vi "fgv_gloabal-config.vi"(7 "cmd":T4, 11 "config_aging":T1 {"Test Specs"."출력단 특성전류 Irms[mA]  Min" format="%#.2f"; "Test Specs"."출력단 특성 전류 Irms[mA]  Max" format="%#.2f"; "Test Specs"."출력단 단선 Irms[mA](이하)" format="%#.2f"; "Test Specs"."제어단 특성 전류 Irms[mA] Min" format="%#.2f"; "Test Specs"."제어단 특성 전류 Irms[mA] Max" format="%#.2f"; "Test Specs"."제어단 단선 Irms[mA](이하)" format="%#.2f"}) -> (3 "config_aging 2":T1 {"Test Specs"."출력단 특성전류 Irms[mA]  Min" format="%#.2f"; "Test Specs"."출력단 특성 전류 Irms[mA]  Max" format="%#.2f"; "Test Specs"."출력단 단선 Irms[mA](이하)" format="%#.2f"; "Test Specs"."제어단 특성 전류 Irms[mA] Min" format="%#.2f"; "Test Specs"."제어단 특성 전류 Irms[mA] Max" format="%#.2f"; "Test Specs"."제어단 단선 Irms[mA](이하)" format="%#.2f"})   [LabVIEW 2019]
uses:
  _ctrl/rw.ctl
  _ctrl/config_aging.ctl
  Register/Setting_reg.ctl
  Breakdown-Spec.ctl
panel:
  # "제어단"
  # "출력단"
  # "온도기준"
  # "Highpower"
  # "Control"
  # "제어단"
  # "출력단"
  # "온도기준"
  # "Highpower"
  # "Control"
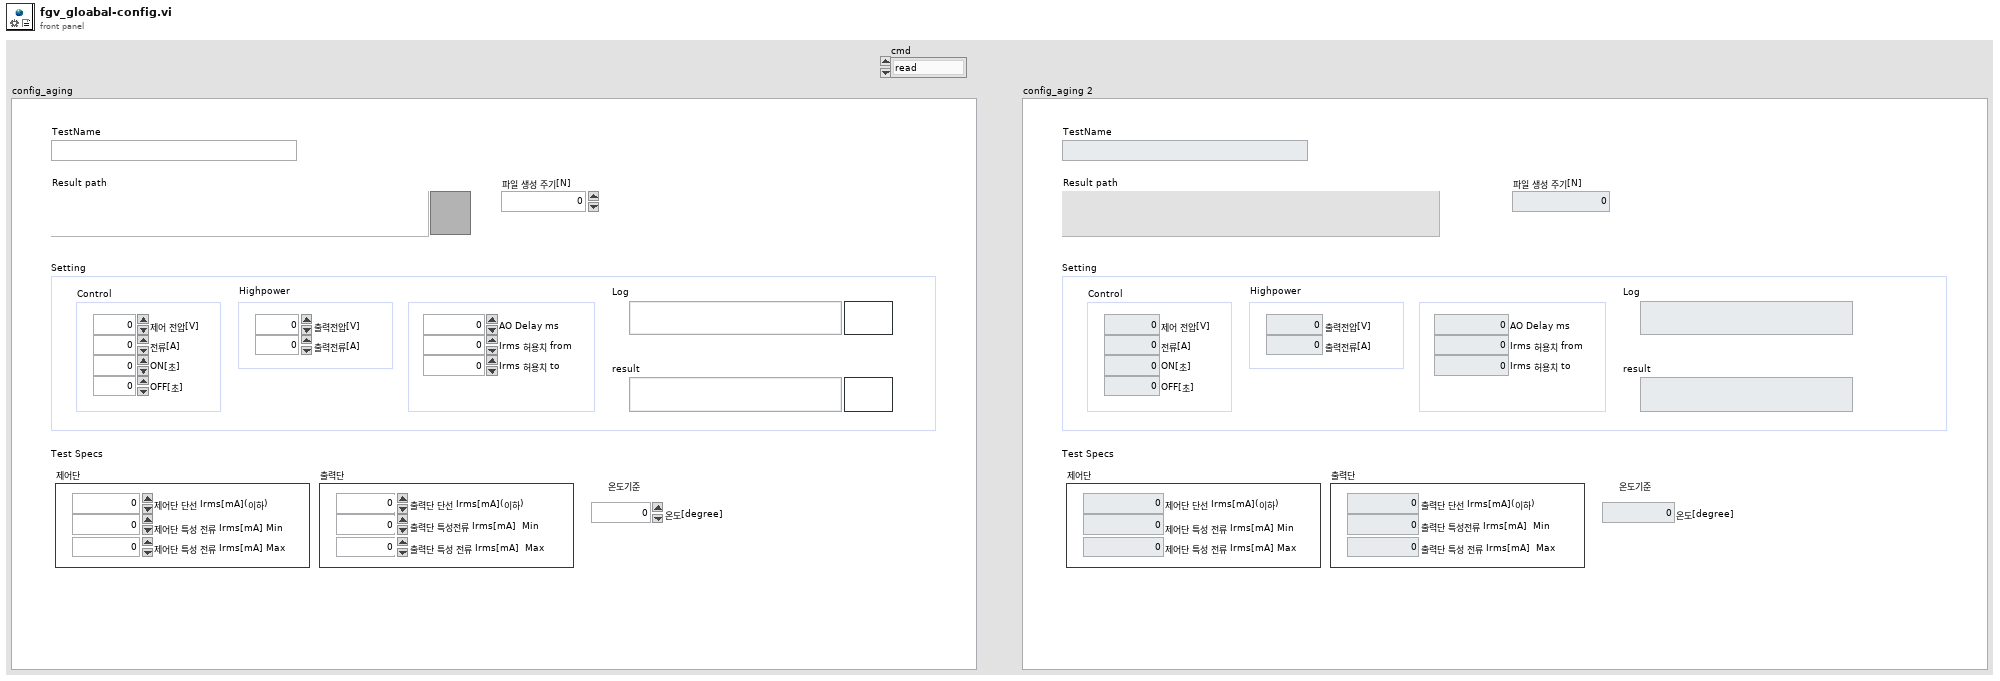
[diagram p1: front panel]
types:
  T1 = typedef "config_aging.ctl" = cluster{"Setting":T2, "TestName":string, "Result path":path, "파일 생성 주기[N]":u8, "Test Specs":T3}
  T2 = typedef "Setting_reg.ctl" = cluster{"제어 전압[V]":dbl, "출력전압[V]":dbl, "전류[A]":dbl, "출력전류[A]":dbl, "ON[초]":dbl, "OFF[초]":dbl, "Irms 허용치 from ":dbl, "Irms 허용치 to":dbl, "AO Delay ms":u32, "Log":path, "result":path}
  T3 = typedef "Breakdown-Spec.ctl" = cluster{"제어단 단선 Irms[mA](이하)":dbl, "제어단 특성 전류 Irms[mA] Max":dbl, "제어단 특성 전류 Irms[mA] Min":dbl, "출력단 단선 Irms[mA](이하)":dbl, "출력단 특성 전류 Irms[mA]  Max":dbl, "출력단 특성전류 Irms[mA]  Min":dbl, "온도[degree]":dbl}
  T4 = typedef "rw.ctl" = enum16{"read", "write"}
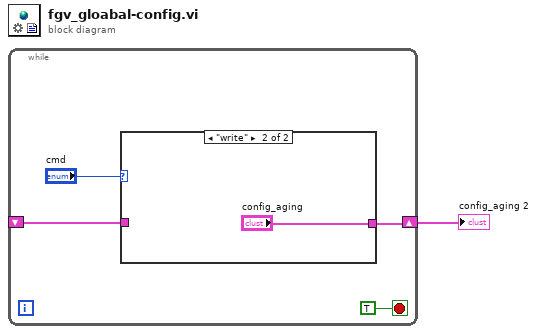
[diagram p0: block diagram]
diagram:
  n1 = while {
    shift-right: [w3] -> w1
    shift-left: _ -> [w2]
    stop <- TRUE stop-if-true
    n2 = case shown="\"write\"" "cmd" {
      tunnel: [w6 "config_aging"] -> w3
      tunnel: w2 -> [w6 _]
      frame "read", Default {
      }
      frame "write" {
      }
    }
  }
  "config_aging 2" <- w1
